vi "Write notifiers.vi"(8 "error in (no error)":errorcluster, 10 "notifier":refnum<notifier>, 11 "Oscilloscope in":refnum<class "Oscilloscope.lvclass">) -> (0 "error out":errorcluster, 3 "Oscilloscope out":refnum<class "Oscilloscope.lvclass">)   [LabVIEW 2015, in "Oscilloscope.lvclass"]
uses:
  Oscilloscope.lvclass
  Oscilloscope.lvclass/Oscilloscope.ctl
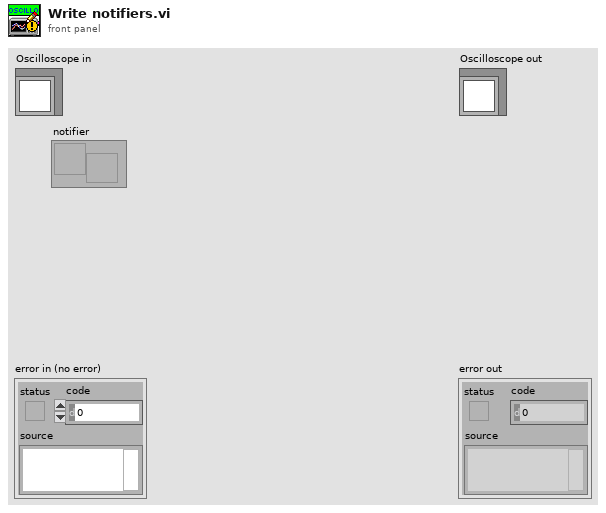
[diagram p1: front panel]
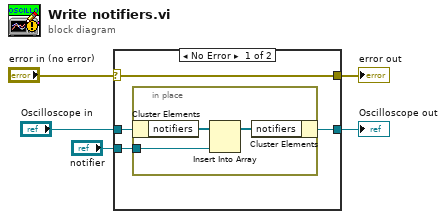
[diagram p0: block diagram]
diagram:
  n1 = case shown="No Error" "error in (no error)" {
    selector: "error in (no error)" -> [w9 w13]
    tunnel: [w9 w13] -> w4
    tunnel: [w7 w14] -> w2
    tunnel: "Oscilloscope in" -> [w8 w14]
    tunnel: "notifier" -> [w6 _]
    frame No Error {
      n2 = in-place {
        in-place-border: w6 -> [w11]
        n3 = in-place-cluster #1(w8) -> ("notifiers"=w12:refnum<notifier>[])
        n4 = Insert Into Array(array=w12, new element=w11) -> (w10:refnum<notifier>[])  [unwired: 1 in]
        n5 = in-place-cluster #1("notifiers"=w10) -> (w7:refnum<class "Oscilloscope.lvclass">)
      }
    }
    frame Error {
    }
  }
  "error out" <- w4
  "Oscilloscope out" <- w2
